vi "tri-state_led.vi"(9 "CLOSE":bool, 10 "OPEN":bool, 11 "ref in":refnum<vi>) -> ()   [LabVIEW 2011]
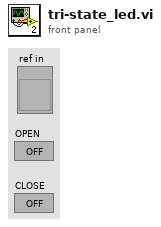
[diagram p1: front panel]
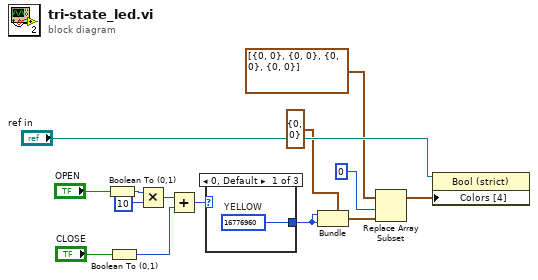
[diagram p0: block diagram]
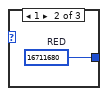
[diagram p2: hidden frame]
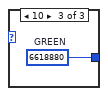
[diagram p3: hidden frame]
diagram:
  n1 = Boolean To (0,1)(Boolean="OPEN") -> (0, 1=w8:i16)
  n2 = Boolean To (0,1)(Boolean="CLOSE") -> (0, 1=w12:i16)
  n3 = Multiply(x=w8, y=i16 10) -> (x*y=w10:i16)
  n4 = Add(x=w10, y=w12) -> (x+y=w11:i16)
  n5 = case shown="0, Default" w11 {
    tunnel: [w15 w16 w17] -> w2
    frame 0, Default {
      w15 = 16776960  # YELLOW
    }
    frame 1 {
      w16 = 16711680  # RED
    }
    frame 10 {
      w17 = 6618880  # GREEN
    }
  }
  n6 = Bundle(cluster=cluster{u32, u32} {0, 0}, w2, w2) -> (w4:cluster{u32, u32})
  n7 = Replace Array Subset(array=cluster{u32, u32}[] [{0, 0}, {0, 0}, {0, 0}, {0, 0}] ("Colors [4]"), new element=w4, index=0) -> (w14:cluster{u32, u32}[])
  n8 = property on="Property Node" class="Bool (strict)"(reference="ref in", "Colors [4]"=w14) -> ()  [unwired: 1 in, 2 out]
